vi "Creds Config Path.vi"() -> (3 "Creds Config Path":path)   [LabVIEW 2020, in "GPack.lvlib" / "GPackPrefs.lvclass"]
uses:
  GPackPrefs.lvclass
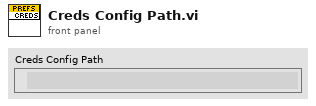
[diagram p1: front panel]
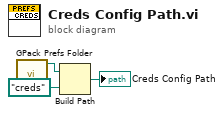
[diagram p0: block diagram]
diagram:
  n1 = call "GPack Prefs Folder.vi"() -> ("GPack Prefs Folder"=w1:path)  [unwired: 10 in, 1 out]
  n2 = Build Path(base path=w1, name or relative path=path "creds") -> (appended path=→"Creds Config Path":path)
